vi "Hann Windows.vi"(8 "error in (no error)":errorcluster, 10 "Window Order":i32, 11 "side points (6)":i32=6) -> (0 "error out":errorcluster, 3 "Window":dbl[](array[numeric]))   [LabVIEW 2019, in "xy_utilities.lvlib"]
uses:
  <vilib>/Analysis/4window.llb/windowTd.ctl
  <vilib>/Analysis/4window.llb/Symmetric Window (DBL).vi
  xy_utilities.lvlib
  <vilib>/Analysis/NI_AALPro.lvlib
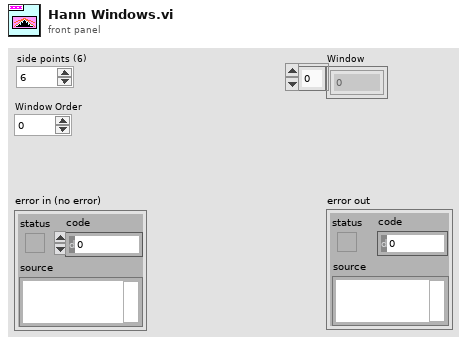
[diagram p1: front panel]
types:
  T1 = typedef "NI_AALPro.lvlib/windowTd.ctl" = u32
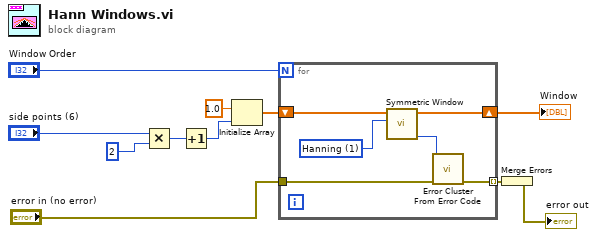
[diagram p0: block diagram]
diagram:
  n1 = Multiply(x="side points (6)", y=2) -> (x*y=w8:i32)
  n2 = Increment(x=w8) -> (x+1=w7:i32)
  n3 = Initialize Array(1.0 ("element"), w7) -> (w6:dbl[])
  n4 = for {
    N: "Window Order" -> [_]
    shift-right: [w15] -> w5
    shift-left: w6 -> [w17]
    tunnel: "error in (no error)" -> [w13]
    tunnel: [w12] -> w2 mode=indexing
    w16 = T1 1 items=["Rectangle"=0, "Hanning"=1, "Hamming"=2, "Blackman-Harris"=3, "Exact Blackman"=4, "Blackman"=5, "Flat Top"=6, "4 Term B-Harris "=7, "7 Term B-Harris"=8, "Low Sidelobe"=9, "Blackman Nuttall"=11, "Triangle"=30, "Bartlett-Hanning"=31, "Bohman"=32, "Parzen"=33, "Welch"=34, "Kaiser"=60, "Dolph-Chebyshev"=61, "Gaussian"=62] ("window")
    n5 = call-poly <vilib>:"Symmetric Window.vi"("window"=w16, "X"=w17) -> ("error"=w14:i32, "Windowed X"=w15:dbl[])  [unwired: 8 in]
    n6 = call <vilib>:"Error Cluster From Error Code.vi"("error in (no error)"=w13, "error code (0)"=w14) -> ("error out"=w12:errorcluster)  [unwired: 7 in]
  }
  "Window" <- w5
  n7 = Merge Errors(w2) -> (→"error out":errorcluster)
